vi "VI.vi"(2 "error in (no error)":errorcluster, 3 "Selector":bool) -> (0 "error out":errorcluster, 1 "Grafica":dbl[](graph))   [LabVIEW 2016]
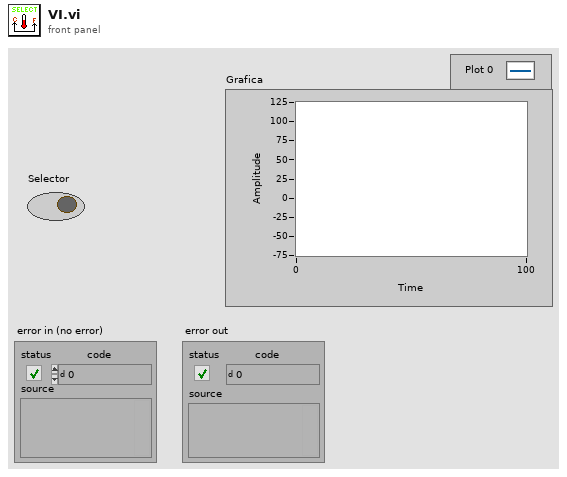
[diagram p1: front panel]
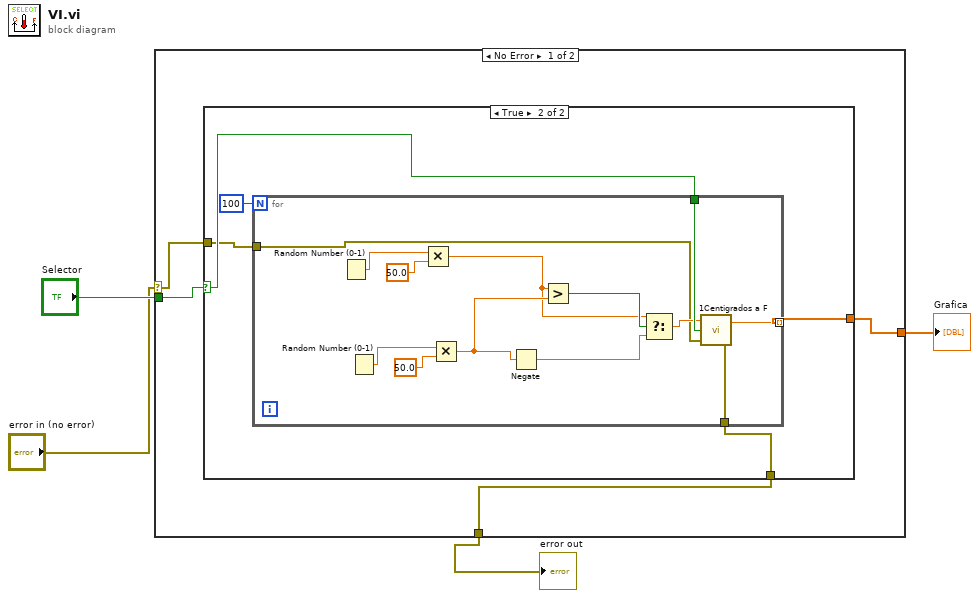
[diagram p0: block diagram]
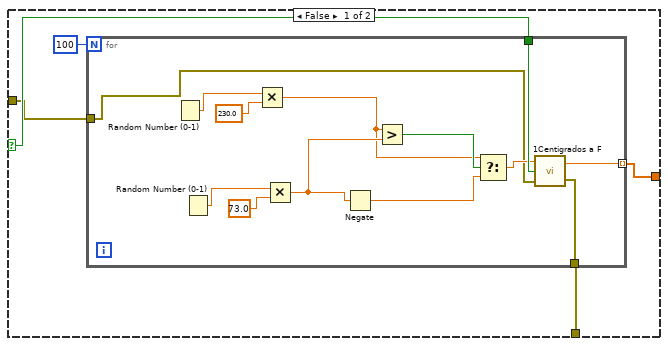
[diagram p2: hidden frame]
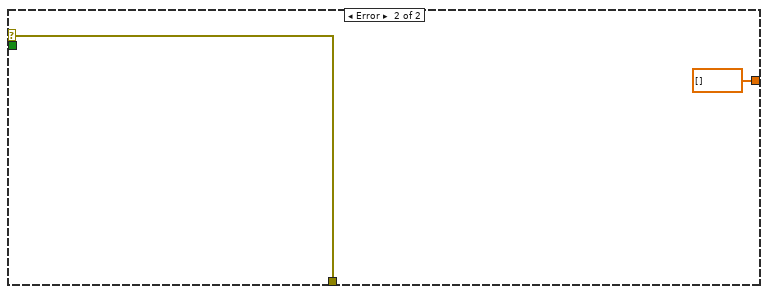
[diagram p3: hidden frame]
diagram:
  n1 = case shown="No Error" "error in (no error)" {
    selector: "error in (no error)" -> [w6 w46]
    tunnel: [w8 dbl[] []] -> w4
    tunnel: "Selector" -> [w7 _]
    tunnel: [w5 w46] -> w1
    frame No Error {
      n2 = case shown="True" w7 {
        selector: w7 -> [w11 w29]
        tunnel: [w12 w30] -> w8
        tunnel: w6 -> [w10 w28]
        tunnel: [w9 w27] -> w5
        frame False {
          n3 = for {
            N: 100 -> [_]
            tunnel: w11 -> [w18]
            tunnel: [w16] -> w12 mode=indexing
            tunnel: w10 -> [w15]
            tunnel: [w14] -> w9
            n4 = Random Number (0-1)() -> (number: 0 to 1=w26:dbl)
            n5 = Random Number (0-1)() -> (number: 0 to 1=w24:dbl)
            n6 = Multiply(x=w26, y=230.0) -> (x*y=w20:dbl)
            n7 = Multiply(x=w24, y=73.0) -> (x*y=w22:dbl)
            n8 = Negate(x=w22) -> (-x=w19:dbl)
            n9 = Greater?(x=w20, y=w22) -> (0:w21:bool)
            n10 = Select(t=w20, s=w21, f=w19) -> (s? t:f=w17:dbl)
            n11 = call "1Centigrados a F.vi"("error in (no error)"=w15, "Selector"=w18, "Temperatura"=w17) -> ("error out"=w14:errorcluster, "Conversion"=w16:dbl)
          }
        }
        frame True {
          n12 = for {
            N: 100 -> [_]
            tunnel: w29 -> [w36]
            tunnel: [w34] -> w30 mode=indexing
            tunnel: w28 -> [w33]
            tunnel: [w32] -> w27
            n13 = Random Number (0-1)() -> (number: 0 to 1=w44:dbl)
            n14 = Random Number (0-1)() -> (number: 0 to 1=w42:dbl)
            n15 = Multiply(x=w44, y=50.0) -> (x*y=w38:dbl)
            n16 = Multiply(x=w42, y=50.0) -> (x*y=w40:dbl)
            n17 = Negate(x=w40) -> (-x=w37:dbl)
            n18 = Greater?(x=w38, y=w40) -> (0:w39:bool)
            n19 = Select(t=w38, s=w39, f=w37) -> (s? t:f=w35:dbl)
            n20 = call "1Centigrados a F.vi"("error in (no error)"=w33, "Selector"=w36, "Temperatura"=w35) -> ("error out"=w32:errorcluster, "Conversion"=w34:dbl)
          }
        }
      }
    }
    frame Error {
    }
  }
  "Grafica" <- w4
  "error out" <- w1
